vi "Sampling Data.vi"(11 "Waveform in":waveform(dbl)) -> (1 "Samples per iteration":dbl, 2 "Sampling frequency":dbl, 3 "Sampling period":dbl, 4 "number of samples":i32)   [LabVIEW 2014, in "Aquisicao de Dados.lvlib"]
uses:
  Aquisicao de Dados.lvlib
  <vilib>/Waveform/WDTOps.llb/WDT Waveform Duration DBL.vi
  <vilib>/Waveform/WDTOps.llb/WDT Number of Waveform Samples DBL.vi
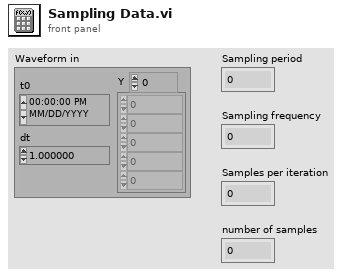
[diagram p1: front panel]
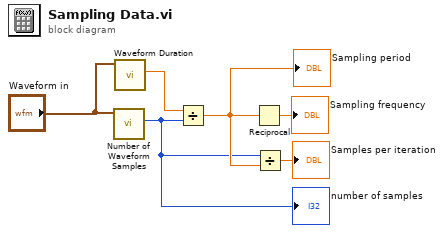
[diagram p0: block diagram]
diagram:
  n1 = call-poly <vilib>:"Number of Waveform Samples.vi"("waveform in"="Waveform in") -> ("number of samples"=w4:i32)  [unwired: 8 in, 2 out]
  "number of samples" <- w4
  n2 = call-poly <vilib>:"Waveform Duration.vi"("waveform in"="Waveform in") -> ("duration"=w2:dbl)  [unwired: 8 in, 2 out]
  n3 = Divide(x=w2, y=w4) -> (x/y=w5:dbl)
  "Sampling period" <- w5
  n4 = Reciprocal(x=w5) -> (1/x=→"Sampling frequency":dbl)
  n5 = Divide(x=w4, y=w5) -> (x/y=→"Samples per iteration":dbl)
